vi "Pre Launch Init.vi"(11 "Example Controller Actor In":refnum<class "Example Controller.lvclass">) -> (0 "Error Out":errorcluster, 3 "Example Controller Actor Out":refnum<class "Example Controller.lvclass">)   [LabVIEW 2023, in "Example GUI View.lvlib" / "Example Controller.lvclass"]
doc: "(<B>Filename</B>: Actor Framework.lvlib:Actor.lvclass:Pre Launch Init.vi)\n\nDefines behavior that occurs after the Launch Nested Actor method is invoked but before the actor's Actor Core method begins running.\n\nBy default, this method does nothing. A descendant class may override it to define behavior."
uses:
  Example Controller.lvclass
  <vilib>/ActorFramework/Message Enqueuer/Message Enqueuer.lvclass
  Example Controller.lvclass/Example Controller.ctl
  Example Controller/Example Controller/Example Controller.lvclass
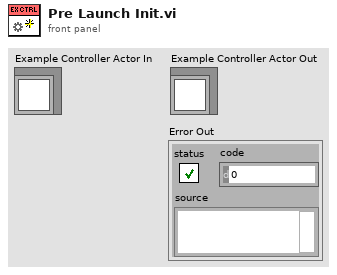
[diagram p1: front panel]
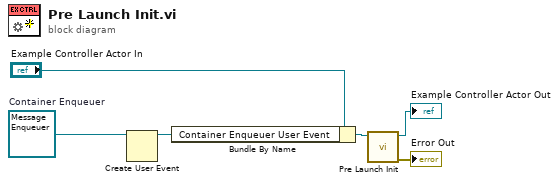
[diagram p0: block diagram]
diagram:
  w3 = refnum<class "Message Enqueuer.lvclass"> refnum  # Container Enqueuer
  n1 = Create User Event(user event datatype=w3) -> (user event=w1:refnum<user-event>)  [unwired: 1 in, 1 out]
  n2 = Bundle By Name(cluster="Example Controller Actor In", "Container Enqueuer User Event"=w1) -> (w2:refnum<class "Example Controller.lvclass">)
  n3 = call-parent "Pre Launch Init.vi"("Controller In"=w2) -> ("Error Out"=→"Error Out":errorcluster, "Controller Out"=→"Example Controller Actor Out":refnum<class "Example Controller.lvclass">)  [unwired: 9 in]
